vi "GetDataType.vi"(8 "error in (no error)":errorcluster, 10 "Channel Number (1-4)":T1=1 items=["Channel 1"=1, "Channel 2"=2, "Channel 3"=3, "Channel 4"=4], 11 "VISA resource name":refnum<visa-resource-name>) -> (0 "error out":errorcluster, 2 "Data Type":string, 3 "VISA resource name out":refnum<visa-resource-name>)   [LabVIEW 2023, in "Thermotron 8800.lvlib"]
doc: "DTYP\nCommand name: Send data type\nCommand type: System status\nDescription: The 8800 sends an integer representing the channel’s data type.\nData type codes:\n0 Unused\n1 Temperature\n2 RH wet bulb/dry bulb\n3 RH linear\n4 RH temperature compensated\n5 Linear\n6 Altitude (kilofeet)\n7 Vibration\n8 Scaled linear\n9 Altitude linear (torr)\n10 Temperature average\n11 Humidity ratio\n12 Dew point\n13 Transducer\n14 Temperature minimum\n15 Temperature maximum\n\nSyntax: DTYPn?\nWhere n is a channel number (1 through 140).\n1 through 8 Process variable channels\n9 through 12 Unused\n13 through 52 Monitor channels 1 - 40\n101 through 140 Monitor channels 1 -40\nData type: Integer\nQuery example: DTYP1?\n8800 response: 1 (The process variable channel 1 data type is temperature.)"
uses:
  Thermotron 8800.lvlib
  Private/AnalogInputChannelNumber 1-4.ctl
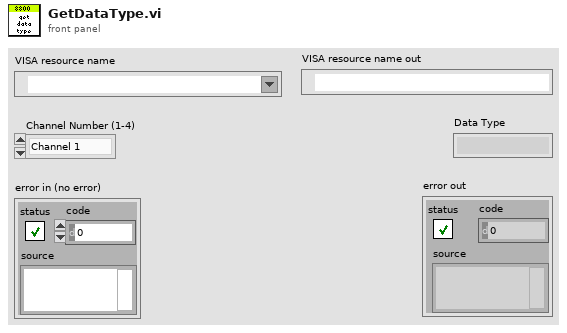
[diagram p1: front panel]
types:
  T1 = typedef "Thermotron 8800.lvlib/AnalogInputChannelNumber 1-4.ctl" = u16
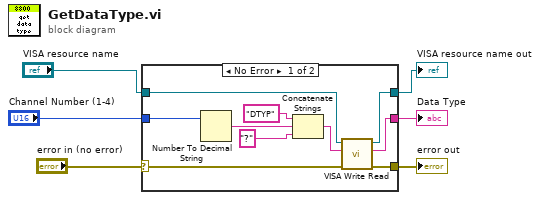
[diagram p0: block diagram]
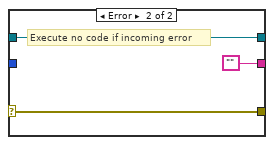
[diagram p2: hidden frame]
diagram:
  n1 = case shown="No Error" "error in (no error)" {
    selector: "error in (no error)" -> [w11 w18]
    tunnel: "Channel Number (1-4)" -> [w10 _]
    tunnel: "VISA resource name" -> [w16 w17]
    tunnel: [w14 w17] -> w5
    tunnel: [w13 ""] -> w4
    tunnel: [w12 w18] -> w3
    frame No Error {
      n2 = Number To Decimal String(number=w10) -> (decimal integer string=w8:string)  [unwired: 1 in]
      n3 = Concatenate Strings("DTYP" ("command"), w8, "?" ("command")) -> (w15:string)
      n4 = call "VISA Write Read.vi"("error in (no error)"=w11, "8800 Command"=w15, "VISA Refnum in"=w16) -> ("error out"=w12:errorcluster, "read buffer"=w13:string, "VISA Refnum out"=w14:refnum<visa-resource-name>)  [unwired: 6 in]
    }
    frame Error {
      # "Execute no code if incoming error"
    }
  }
  "VISA resource name out" <- w5
  "error out" <- w3
  "Data Type" <- w4
